vi "PH_SSAC.allocate or free img space.vi"(0 "i ref in":refnum<vi>, 2 "Allocate?":bool, 5 "error in (no error)":errorcluster) -> (14 "i ref out":refnum<vi>, 19 "error out":errorcluster)   [LabVIEW 2014, in "PH_SSAC.lvlib"]
doc: "This VI is forseen to be used in constructor or destructor. If Allocate? = true is chosen, memory space for several images is allocated. If false is chosen, it is freed."
uses:
  PH_SSAC.lvlib
  CS_Core/CSSystem/CSSystemLib/CSSystemLib.lvlib
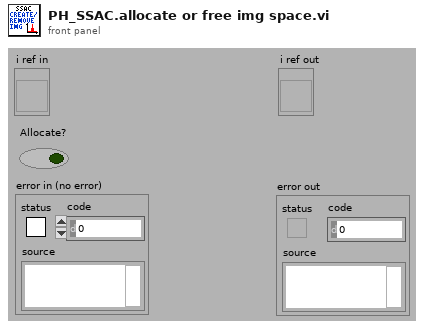
[diagram p1: front panel]
types:
  T1 = typedef "PH_SSAC.lvlib/PH_SSAC.i attribute.ctl" = cluster{"GUI Refs":cluster{"Delete":refnum<vi>, "Global On":refnum<vi>, "Cam Source":refnum<vi>, "Frame Main Signal":refnum<vi>, "Frame Background":refnum<vi>, "dt (Gauss smooth)":refnum<vi>, "Calibration Factor":refnum<vi>, "Background acquire":refnum<vi>, "Threshold":refnum<vi>, "Time evolution of mean pulse duration":refnum<vi>, "Mean Pulse Duration":refnum<vi>, "Main signal":refnum<vi>, "Current Pulse Duration":refnum<vi>, "Processed":refnum<vi>, "Saturation":refnum<vi>, "# for Average":refnum<vi>, "Position":refnum<vi>, "BG Status":refnum<vi>, "Save BG data":refnum<vi>, "Read BG Data":refnum<vi>, "Background Calibration Data":refnum<vi>}, "Images":cluster{"OP Image":T2, "GUI Image":T2, "PSDB Image":T2}, "Global On?":bool, "Frame Main":cluster{"x":u32, "dx":u32, "y":u32, "dy":u32}, "Frame Background":cluster{"x":u32, "dx":u32, "y":u32, "dy":u32}, "dt [fs]":dbl, "Calibration Factor [fs/pixel]":dbl, "Threshold":dbl, "Time evolution of mean pulse duration [fs]":dbl[], "Main Signal":cluster{"Time for Main":dbl[], "Signal":dbl[]}, "Processed":bool, "Current Pulse Duration [fs]":dbl, "# for Average":i32, "Position":i32, "Pulse Durations [fs]":dbl[], "BG":cluster{"Acquire?":bool, "Background Calibration Data":T3, "Save Data":bool}}
  T2 = typedef "IMAQ Image.ctl" = refnum<image>
  T3 = typedef "PH_SSAC.lvlib/PH_SSAC.Background Data.ctl" = cluster{"Date":string, "Time":string, "Frame Main":cluster{"x":u32, "dx":u32, "y":u32, "dy":u32}, "dt [fs]":dbl, "Calibration Factor [fs/pixel]":dbl, "Signal":dbl[], "Frame Background":cluster{"x":u32, "dx":u32, "y":u32, "dy":u32}}
  T4 = cluster{"OP Image":T2, "GUI Image":T2, "PSDB Image":T2}
  T5 = typedef "Image Type" = u32
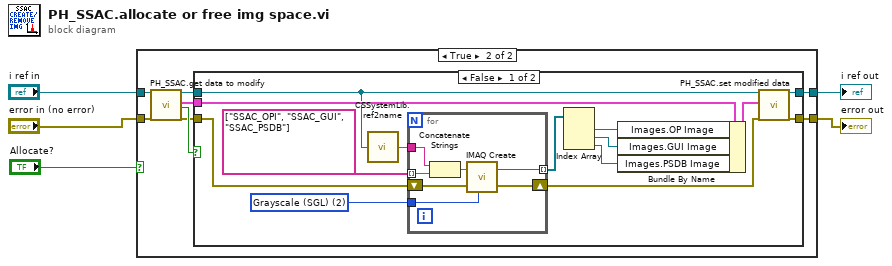
[diagram p0: block diagram]
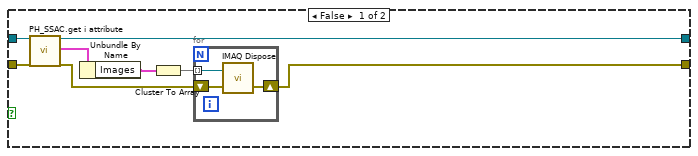
[diagram p2: hidden frame]
diagram:
  n1 = case shown="True" "Allocate?" {
    tunnel: [w8 w23] -> w5
    tunnel: [w10 w22] -> w4
    tunnel: "error in (no error)" -> [w13 w19]
    tunnel: "i ref in" -> [w12 w18]
    frame False {
      n2 = call "PH_SSAC.get i attribute.vi"("i ref in"=w12, "error in (no error)"=w13) -> ("i ref out"=w10:refnum<vi>, "i attribute"=w11:T1, "error out"=w9:errorcluster)  [unwired: 15 in]
      n3 = Unbundle By Name(w11) -> ("Images"=w7:T4)
      n4 = Cluster To Array(cluster=w7) -> (array=w6:T2[])
      n5 = for {
        shift-right: [w15] -> w8
        shift-left: w9 -> [w16]
        tunnel: w6 -> [w14] mode=indexing
        n6 = call "IMAQ Dispose"("Image"=w14, "error in (no error)"=w16) -> ("error out"=w15:errorcluster)  [unwired: 4 in]
      }
    }
    frame True {
      n7 = call "PH_SSAC.get data to modify.vi"("i ref in"=w18, "error in (no error)"=w19) -> ("i ref out"=w21:refnum<vi>, "i attribute"=w17:T1, "timed out"=w24:bool, "error out"=w20:errorcluster)  [unwired: 14 in]
      n8 = case shown="False" w24 {
        tunnel: w20 -> [w33 w46]
        tunnel: w21 -> [w29 w47]
        tunnel: [w38 w47] -> w22
        tunnel: [w37 w46] -> w23
        tunnel: w17 -> [w36 _]
        frame False {
          w30 = T5 2 items=["Grayscale (U8)", "Grayscale (I16)", "Grayscale (SGL)", "Complex (CSG)", "RGB (U32)", "HSL (U32)", "RGB (U64)"] ("Image Type")
          n9 = call "CSSystemLib.ref2name.vi"("obj refnum"=w29) -> ("name"=w28:string)
          n10 = for {
            shift-right: [w45] -> w34
            shift-left: w33 -> [w44]
            tunnel: [w39] -> w32 mode=indexing
            tunnel: string[] ["SSAC_OPI", "SSAC_GUI", "SSAC_PSDB"] -> [w41] mode=indexing
            tunnel: w30 -> [w43]
            tunnel: w28 -> [w42]
            n11 = Concatenate Strings(w42, w41) -> (w40:string)
            n12 = call "IMAQ Create"("Image Name"=w40, "Image Type"=w43, "error in (no error)"=w44) -> ("New Image"=w39:T2, "error out"=w45:errorcluster)  [unwired: 2 in]
          }
          n13 = Index Array(array=w32) -> (element #1=w27:T2, element #2=w26:T2, element #3=w25:T2)  [unwired: 3 in]
          n14 = Bundle By Name(cluster=w36, "Images.OP Image"=w27, "Images.GUI Image"=w26, "Images.PSDB Image"=w25) -> (w35:T1)
          n15 = call "PH_SSAC.set modified data.vi"("i ref in"=w29, "i attribute"=w35, "error in (no error)"=w34) -> ("i ref out"=w38:refnum<vi>, "error out"=w37:errorcluster)  [unwired: 15 in]
        }
        frame True {
        }
      }
    }
  }
  "error out" <- w5
  "i ref out" <- w4
